vi "ExSubToggleFlat.vi"(2 "error in (no error)":errorcluster, 3 "Camera Handle":u32) -> (0 "error out":errorcluster, 1 "Camera Handle":u32)   [LabVIEW 2010]
uses:
  GlobalIFlatImgHndl.vi
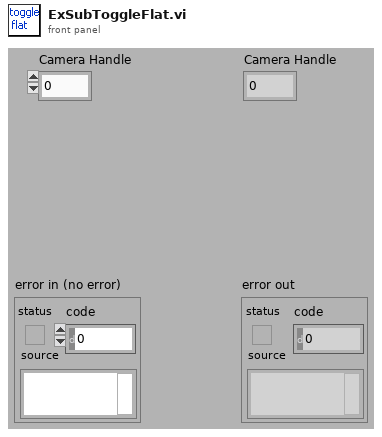
[diagram p1: front panel]
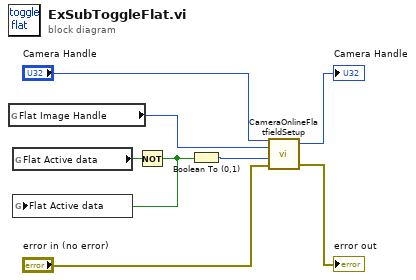
[diagram p0: block diagram]
diagram:
  n1 = global read "GlobalIFlatImgHndl.vi" "Flat Image Handle"() -> (w5:u32)
  n2 = global read "GlobalIFlatImgHndl.vi" "Flat Active data"() -> (w8:bool)
  n3 = Not(x=w8) -> (.not. x?=w7:bool)
  n4 = global write "GlobalIFlatImgHndl.vi" "Flat Active data"(w7) -> ()
  n5 = Boolean To (0,1)(Boolean=w7) -> (0, 1=w6:i16)
  n6 = call <userlib>:"CameraOnlineFlatfieldSetup.vi"("error in"="error in (no error)", "Flat Field Flag"=w6, "Flat Field Image Handle"=w5, "Camera Handle"="Camera Handle") -> ("error out"=→"error out":errorcluster, "Camera Handle"=→"Camera Handle":u32)  [unwired: 1 out]
